vi "845x_I2C Read.vi"(0 "Device":T1, 1 "I/O Voltage Level":i32(ring)=33 items=["3.3V"=33, "2.5V"=25, "1.8V"=18, "1.5V"=15, "1.2V"=12], 2 "Use Internal I2C Pullup Resistor":bool, 5 "Address":u16=80 format="%.0x", 7 "Clock Rate (kHz)":u16=100, 9 "EEPROM Data Address":u16 format="%.0x", 11 "error in (no error)":errorcluster, 12 "Number of Bytes to Read":u32=128 max=65536 step=1, 13 "Data Address Width":enum16{"1 Byte", "2 Byte"}(ring)=enum."2 Byte", 14 "Data Address Endianness":bool=TRUE) -> (4 "Read Data":u8[](array[numeric]) format="%x", 15 "error out":errorcluster)   [LabVIEW 2021, in "Communication.lvlib"]
doc: "<B>NOTE: This example is taken from ni845x driver examples located at C:\\Program Files (x86)\\National Instruments\\LabVIEW <version>\\examples\\ni845x\\845xEx.llb. More such examples can be found in the same location.</B>\n\nThis EEPROM example shows a more generalized way to use the I2C basic API to read data. It allows the user to change the following parameters: the endianness of the address bytes, and the number of bytes in an address.\n\nThe parameters will have the following effects:\n\nData Address Width: This will allow the user to specify the EEPROM Data Address as either 1 or 2 bytes.\nData Address Endianness: This control will change the ordering of the bytes in the EEPROM Data Address, note that this only has an effect if there are 2 bytes in the address.\n\nSince the I2C SDA and SCL lines are open-drain, they must be pulled up to the required reference voltage of your slave by connecting an appropriate resistor (2k-5k) between SCL and your reference voltage and SDA and your reference voltage. For NI-845x Hardware that contain internal pull-ups, you can use these. Otherwise, you need to use external pullups.\n\nFor connection information see the NI-845x Hardware and Software manual and the manual for your specific EEPROM."
uses:
  Communication.lvlib
  <vilib>/ni845x/ni845x.llb/ni845xControl.ctl
  <vilib>/ni845x/ni845x.llb/NI-845x I2C Close Configuration Reference.vi
  <resource>/objmgr/NI845x.rc
panel:
  # "See VI Info <Ctrl+I> for more information on how to use this example"
  # "I2C Data"
  # "Device Configuration"
  # "I2C Slave Configuration"
  # "Big Endian"
  # "Little Endian"
  # "NOTE: This example is taken from ni845x driver examples located at C:\\Program Files (x86)\\National Instruments\\LabVIEW <version>\\examples\\ni845x\\845xEx.llb. More such examples can be found in the same location."
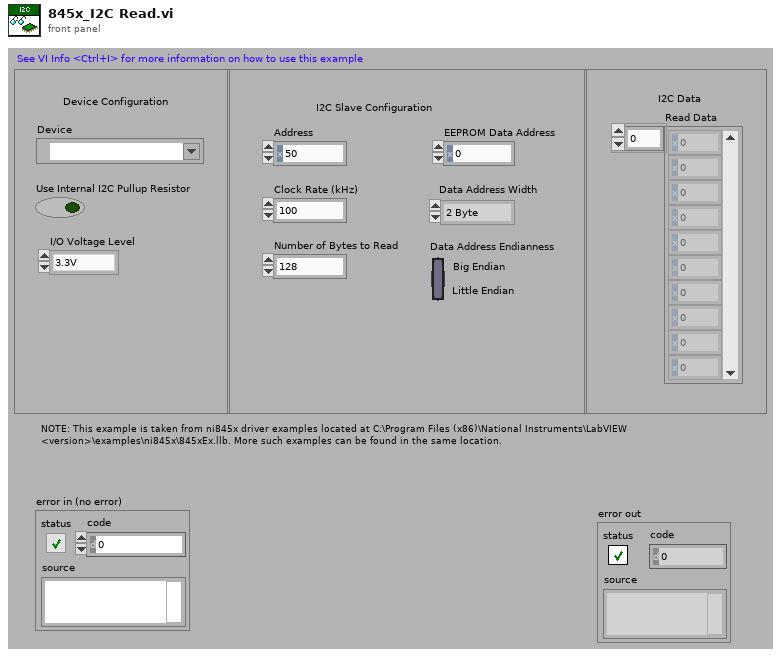
[diagram p1: front panel]
types:
  T1 = typedef "ni845xControl.ctl" = refnum<k21>
  T2 = typedef "ni845xI2cConfiguration.ctl" = refnum<k20>
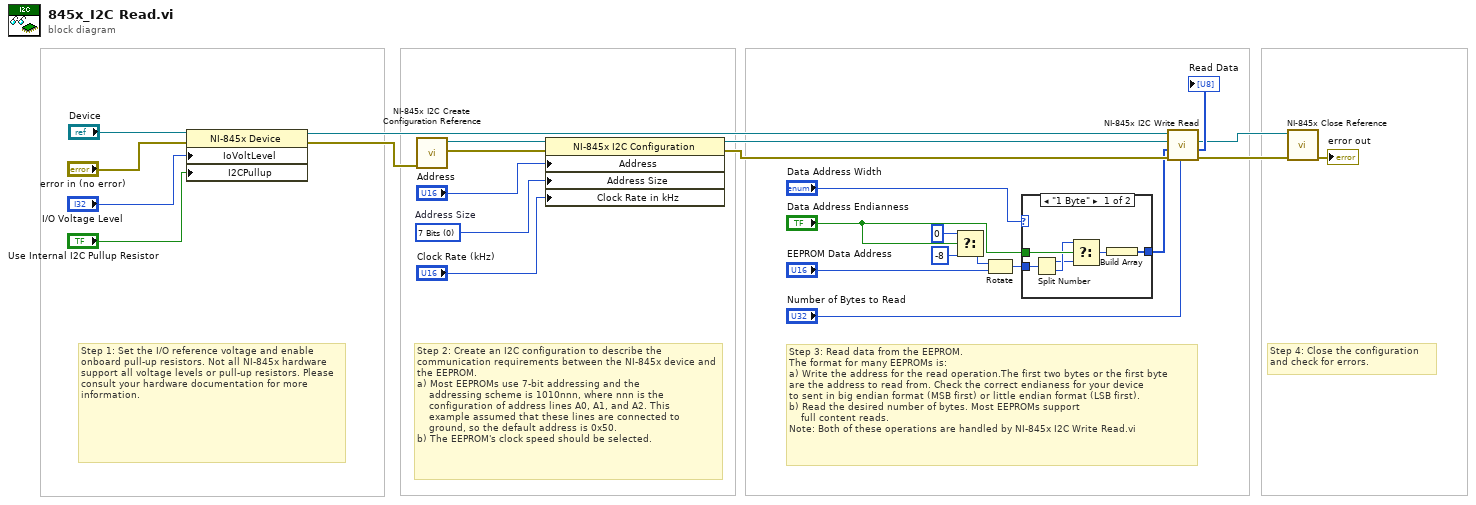
[diagram p0: block diagram]
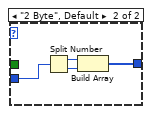
[diagram p2: hidden frame]
diagram:
  w22 = 0 items=["7 Bits", "10 Bits"]  # Address Size
  # "Step 1: Set the I/O reference voltage and enable onboard pull-up resistors. Not all NI-845x hardware support all voltage levels or pull-up resistors. Please consult your hardware documentation for more information."
  # "Step 4: Close the configuration \nand check for errors."
  # "Step 2: Create an I2C configuration to describe the \ncommunication requirements between the NI-845x device and the EEPROM.\na) Most EEPROMs use 7-bit addressing and the\n    addressing scheme is 1010nnn, where nnn is the\n    configuration of address lines A0, A1, and A2. This    \n    example assumed that these lines are connected to\n    ground, so the default address is 0x50. \nb) The EEPROM's clock speed should be selected."
  # "Step 3: Read data from the EEPROM. \nThe format for many EEPROMs is:\na) Write the address for the read operation.The first two bytes or the first byte \nare the address to read from. Check the correct endianess for your device \nto sent in big endian format (MSB first) or little endian format (LSB first).\nb) Read the desired number of bytes. Most EEPROMs support\n    full content reads.  \nNote: Both of these operations are handled by NI-845x I2C Write Read.vi"
  n1 = property on="Property Node" class="NI-845x Device"(reference="Device", error in="error in (no error)", "IoVoltLevel"="I/O Voltage Level", "I2CPullup"="Use Internal I2C Pullup Resistor") -> (reference out=w6:T1, error out=w3:errorcluster)
  n2 = call <vilib>:"NI-845x I2C Create Configuration Reference.vi"("error in (no error)"=w3) -> ("error out"=w19:errorcluster, "i2c configuration"=w20:T2)  [unwired: 9 out]
  n3 = property class="NI-845x I2C Configuration"(reference=w20, error in=w19, "Address"="Address", "Address Size"=w22, "Clock Rate in kHz"="Clock Rate (kHz)") -> (reference out=w25:T2, error out=w24:errorcluster)
  n4 = Select(t=i16 0, s="Data Address Endianness", f=i16 -8) -> (s? t:f=w14:i16)
  n5 = Rotate(1:"EEPROM Data Address", 2:w14) -> (0:w11:u16)
  n6 = case shown="\"1 Byte\"" "Data Address Width" {
    tunnel: [w32 w36] -> w12
    tunnel: w11 -> [w31 w33]
    tunnel: "Data Address Endianness" -> [w29 _]
    frame "1 Byte" {
      n7 = Split Number(x=w31) -> (hi(x)=w27:u8, lo(x)=w28:u8)
      n8 = Select(t=w28, s=w29, f=w27) -> (s? t:f=w30:u8)
      n9 = Build Array(w30) -> (w32:u8[])
    }
    frame "2 Byte", Default {
      n10 = Split Number(x=w33) -> (hi(x)=w35:u8, lo(x)=w34:u8)
      n11 = Build Array(w35, w34) -> (w36:u8[])
    }
  }
  n12 = call <vilib>:"NI-845x I2C Write Read.vi"("num bytes to read"="Number of Bytes to Read", "error in (no error)"=w24, "write data"=w12, "i2c configuration in"=w25, "device reference in"=w6) -> ("error out"=w18:errorcluster, "read data"=→"Read Data":u8[], "i2c configuration out"=w9:T2)  [unwired: 4 out]
  n13 = call-poly <vilib>:"NI-845x Close Reference.vi"("error in (no error)"=w18, "i2c configuration"=w9) -> ("error out"=→"error out":errorcluster)  [unwired: 9 out]
